vi "sc_adjustMotion.vi"(8 "error in (no error)":errorcluster, 9 "speed of descent (finding slice surface)":dbl, 10 "motion":T1=enum."fast", 11 "VISA handle":refnum<visa-resource-name>) -> (0 "error out":errorcluster, 3 "Dup. VISA handle":refnum<visa-resource-name>)   [LabVIEW 2019]
uses:
  controls/scope_motion.ctl
  pipette cleaning/pressure box/cleaning_soft/controls/scientifica_commands.ctl
panel:
  # "DEBUG: FAST AND SLOW SPEEDS ARE THE SAME!! CHANGE THIS"
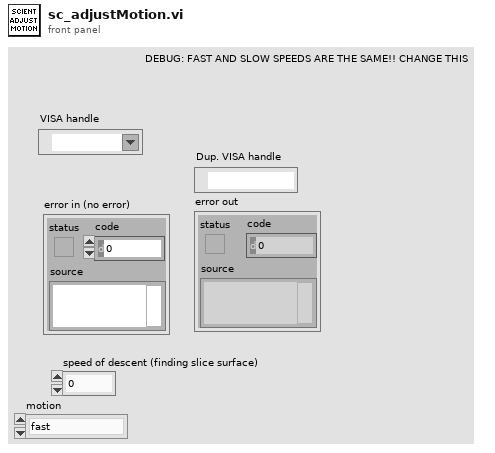
[diagram p1: front panel]
types:
  T1 = typedef "scope_motion.ctl" = enum16{"superSlow", "fast", "slow", "find slice speed", "slow_dualPatch"}
  T2 = typedef "scientifica_commands.ctl" = enum16{"ANGLE", "INSET", "FIRST", "ZERO", "Pz", "P", "absz", "ACC", "TOP", "STOP", "rel", "relz", "abs", "IN", "vj", "APROACH", "OBJS", "OBJU", "OUT", "OBJ", "OBJL", "SET", "OBJD", "STEP", "SETSTEP", "S", "UUX", "UUY", "UUZ"}
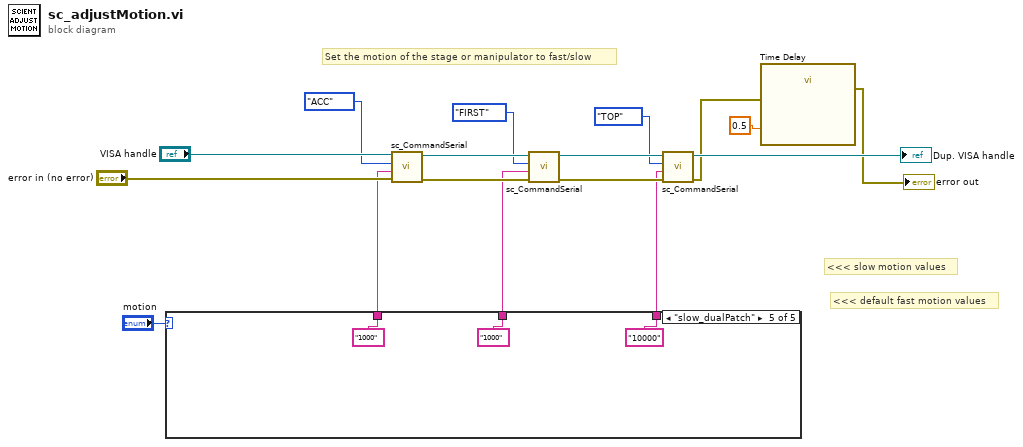
[diagram p0: block diagram]
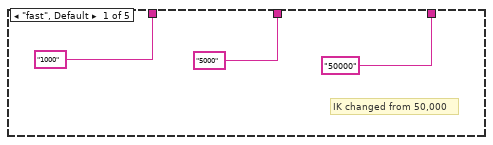
[diagram p2: hidden frame]
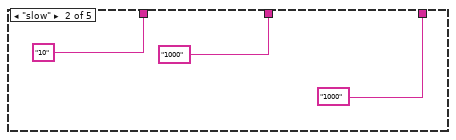
[diagram p3: hidden frame]
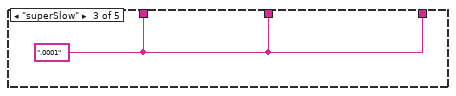
[diagram p4: hidden frame]
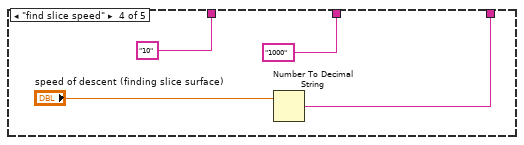
[diagram p5: hidden frame]
diagram:
  # "<<< default fast motion values"
  # "<<< slow motion values"
  # "Set the motion of the stage or manipulator to fast/slow"
  n1 = case shown="\"slow_dualPatch\"" "motion" {
    tunnel: ["1000" "10" w24 "10" "1000"] -> w7
    tunnel: ["5000" "1000" w24 "1000" "1000"] -> w6
    tunnel: ["50000" "1000" ("t") w24 w25 "10000" ("t")] -> w5
    frame "fast", Default {
      # "IK changed from 50,000"
    }
    frame "slow" {
    }
    frame "superSlow" {
      w24 = ".0001"
    }
    frame "find slice speed" {
      n2 = Number To Decimal String(number="speed of descent (finding slice surface)") -> (decimal integer string=w25:string)  [unwired: 1 in]
    }
    frame "slow_dualPatch" {
    }
  }
  n3 = call "sc_CommandSerial.vi"("error in (no error)"="error in (no error)", "argument"=w7, "Scientifica commands"=scientifica_commands."ACC", "VISA handle"="VISA handle") -> ("error out"=w11:errorcluster, "Dup. VISA handle"=w14:refnum<visa-resource-name>)  [unwired: 4 in, 2 out]
  n4 = call "sc_CommandSerial.vi"("error in (no error)"=w11, "argument"=w6, "Scientifica commands"=scientifica_commands."FIRST", "VISA handle"=w14) -> ("error out"=w12:errorcluster, "Dup. VISA handle"=w13:refnum<visa-resource-name>)  [unwired: 4 in, 2 out]
  n5 = call "sc_CommandSerial.vi"("error in (no error)"=w12, "argument"=w5, "Scientifica commands"=scientifica_commands."TOP", "VISA handle"=w13) -> ("error out"=w3:errorcluster, "Dup. VISA handle"=→"Dup. VISA handle":refnum<visa-resource-name>)  [unwired: 4 in, 2 out]
  n6 = call "Time Delay"("error in (no error)"=w3, "Delay Time (s)"=0.5) -> ("error out"=→"error out":errorcluster)  [unwired: 9 in]
